vi "myRIO_BRig_Host_comm_webdav_testConnect.vi"() -> (2 "output_Iconnected":bool)   [LabVIEW 2014]
uses:
  <vilib>/WebDAVClient/NI_WebDAV.lvlib
panel:
  out "code":u8
  out "error out":errorcluster
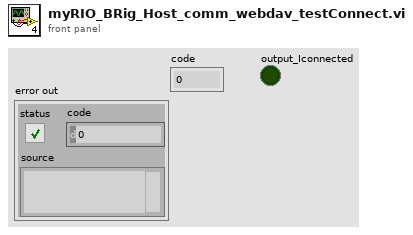
[diagram p1: front panel]
types:
  T1 = typedef "NI_WebDAV.lvlib/SessionHandle.ctl" = refnum<k1>
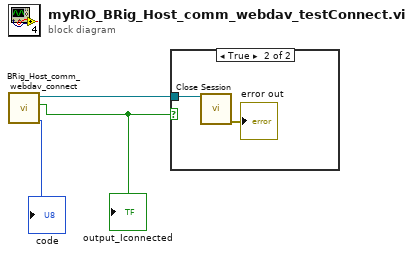
[diagram p0: block diagram]
diagram:
  n1 = call "BRig_Host_comm_webdav_connect.vi"() -> ("output_code"=→"code":u8, "output_Iconnected"=w2:bool, "output_hSession"=w3:T1)  [unwired: 9 in]
  "output_Iconnected" <- w2
  n2 = case shown="True" w2 {
    tunnel: w3 -> [_ w5]
    frame False {
    }
    frame True {
      n3 = call <vilib>:"Close Session.vi"("session handle"=w5) -> ("error out"=→"error out":errorcluster)  [unwired: 14 in]
    }
  }
